vi "testRPM1.vi"() -> ()   [LabVIEW 2014]
uses:
  <vilib>/Analysis/NI_AALBase.lvlib
  <vilib>/Analysis/baseanly.llb/Mean (DBL).vi
panel:
  in  "High Base Speed":dbl
  in  "Low Base speed":dbl
  in  "Fator":dbl
  out "Velocidade(km_h)":dbl
  out "RPM":dbl
  out "Frequency (RPM)":dbl
  out "Filtered Signal 2":dynamicdata(graph) caption="Filtered Signal"
  out "error out":errorcluster
  in  "stop":bool
  out "Frequency":dbl
  out "Raw Signal":dynamicdata(graph) caption="Filtered Signal"
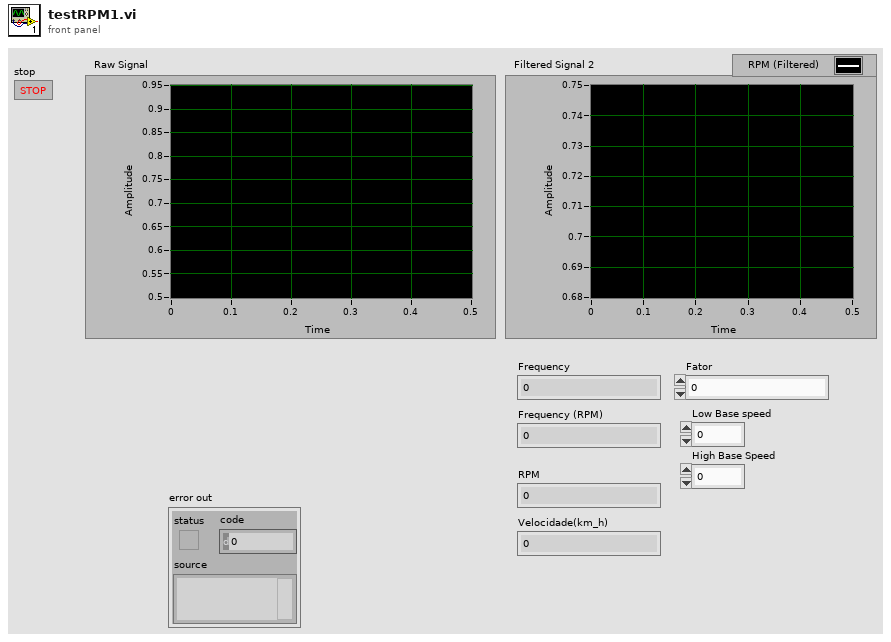
[diagram p1: front panel]
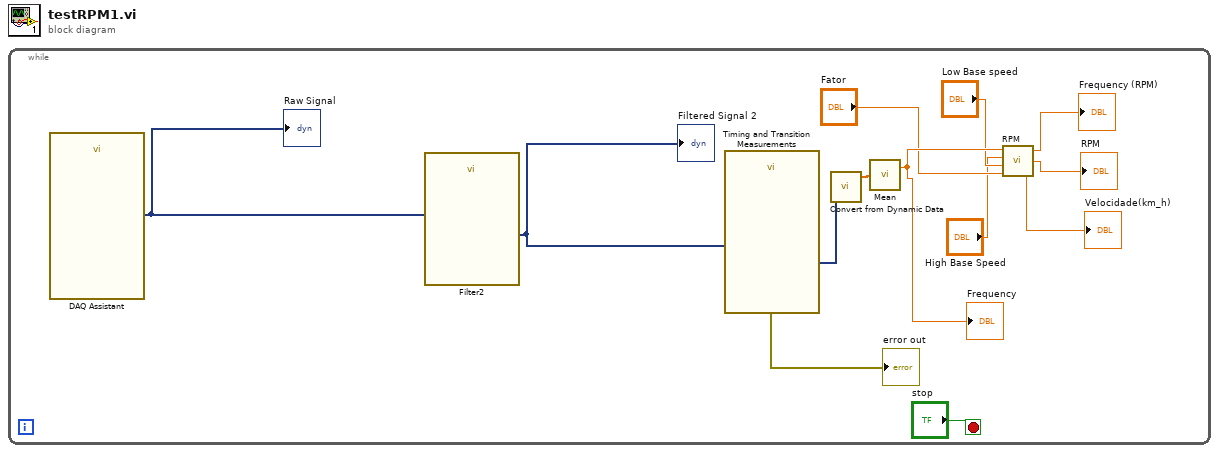
[diagram p0: block diagram]
diagram:
  n1 = while {
    stop <- "stop" stop-if-true
    n2 = call "DAQ Assistant"() -> ("data"=w8:dynamicdata)  [unwired: 16 in, 3 out]
    "Raw Signal" <- w8
    n3 = call "Filter2"("Signal"=w8) -> ("Filtered Signal"=w11:dynamicdata)  [unwired: 9 in, 1 out]
    "Filtered Signal 2" <- w11
    n4 = call "Timing and Transition Measurements"("Signals"=w11) -> ("error out"=→"error out":errorcluster, "Frequency"=w10:dynamicdata)  [unwired: 9 in]
    n5 = call "Convert from Dynamic Data"("Dynamic Data Type"=w10) -> ("Array"=w9:dbl[])  [unwired: 3 in]
    n6 = call-poly <vilib>:"Mean.vi"("X"=w9) -> ("mean"=w4:dbl)  [unwired: 1 out]
    "Frequency" <- w4
    n7 = call "RPM.vi"("factor"="Fator", 4:"Low Base speed", 5:"High Base Speed", "data"=w4) -> ("km/h"=→"Velocidade(km_h)":dbl, "RPM"=→"RPM":dbl, "Frequency"=→"Frequency (RPM)":dbl)
  }
